vi "Configure VF Device Selection.vi"(10 "VF DeviceID":T1, 11 "VF Device Selection in":refnum<class "VF Device Selection.lvclass">) -> (3 "VF Device Selection out":refnum<class "VF Device Selection.lvclass">)   [LabVIEW 2018, in "VF Device Selection Actor.lvlib" / "VF Device Selection.lvclass"]
uses:
  VF Device Selection.lvclass
  <vilib>/ORNL/CSEISMIC DDS/CSEISMIC DDS Base/Data Types/Controls/DeviceID.ctl
  VF Device Selection.lvclass/VF Device Selection.ctl
  <vilib>/ORNL/CSEISMIC DDS/CSEISMIC DDS Base/CSEISMIC DDS.lvclass
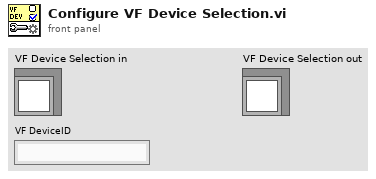
[diagram p1: front panel]
types:
  T1 = typedef "CSEISMIC DDS.lvlib/CSEISMIC DDS.lvclass/DeviceID.ctl" = string
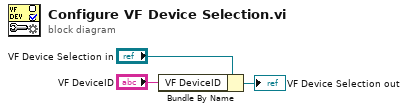
[diagram p0: block diagram]
diagram:
  n1 = Bundle By Name(cluster="VF Device Selection in", "VF DeviceID"="VF DeviceID") -> (→"VF Device Selection out":refnum<class "VF Device Selection.lvclass">)
